vi "shared data GUI.vi"(0 "data update interval":refnum<vi>, 1 "Scroll Refnum":refnum<vi>, 5 "shared folder":refnum<vi>, 9 "My data to share":refnum<vi>, 11 "error in (no error)":errorcluster, 12 "command":enum16{"Initialize", "Update GUI"}(ring), 13 "Write":refnum<vi>, 14 "List of available data":refnum<vi>) -> (4 "Available shared data":T1 {"Shared Data"."scaled" format="%.2f"}, 6 "My data to share":T2 {"scaled" format="%.2f"}, 10 "Cumulative shared data sizes":i32[](array[numeric]), 15 "error out":errorcluster)   [LabVIEW 2015]
uses:
  shared data (name value unit).ctl
  available share data.ctl
  share data command.ctl
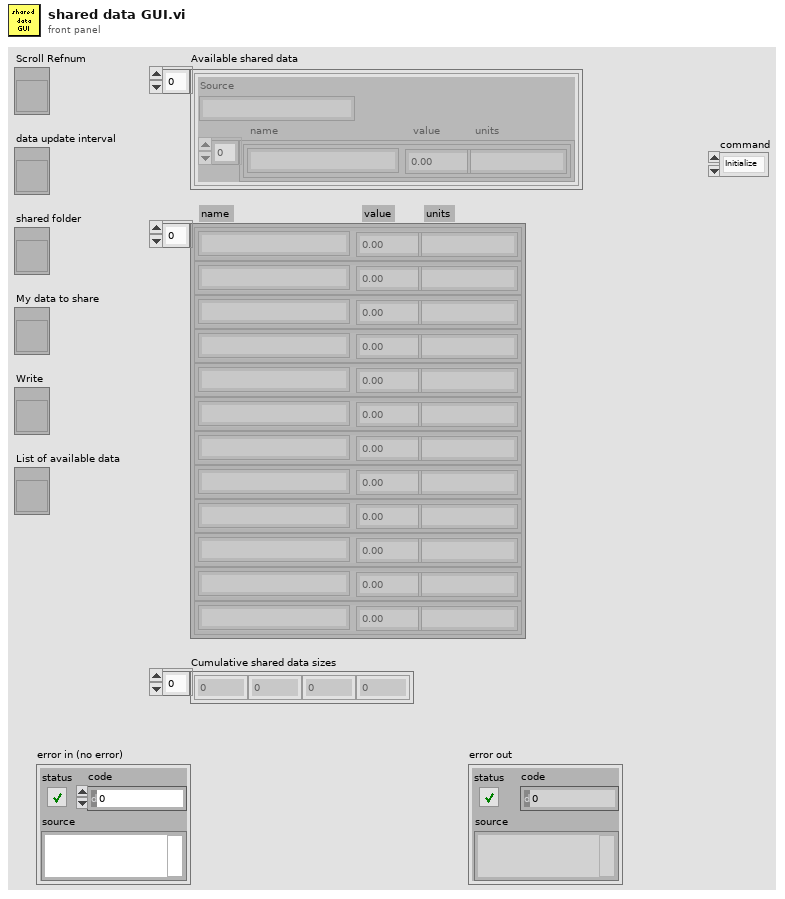
[diagram p1: front panel]
types:
  T1 = typedef "available share data.ctl" = cluster{"Source":string, "Shared Data":T2}[]
  T2 = typedef "shared data (name value unit).ctl" = cluster{"name":string, "units":string, "scaled":sgl}[]
  T3 = typedef "share data command.ctl" = enum16{"Initialize from ini", "Update ini", "Write data", "Read data", "List my data", "List shared data", "Close"}
  T4 = typedef "write data cluster.ctl" = cluster{"Data interval (s)":sgl, "Shared Folder":path, "Write":bool[]}
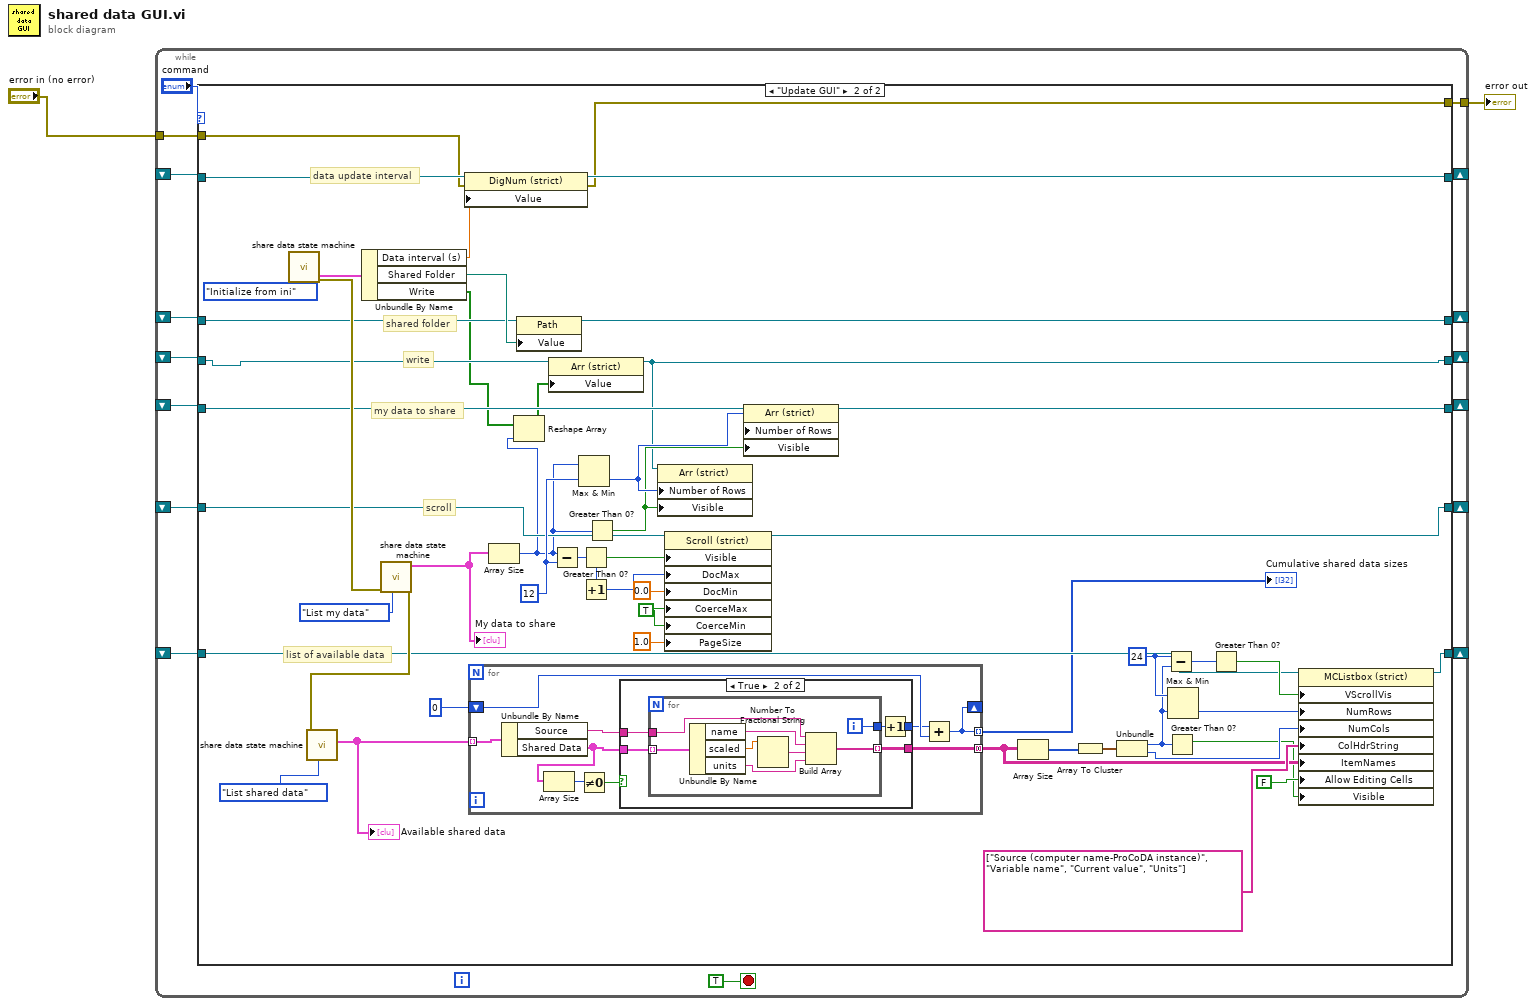
[diagram p0: block diagram]
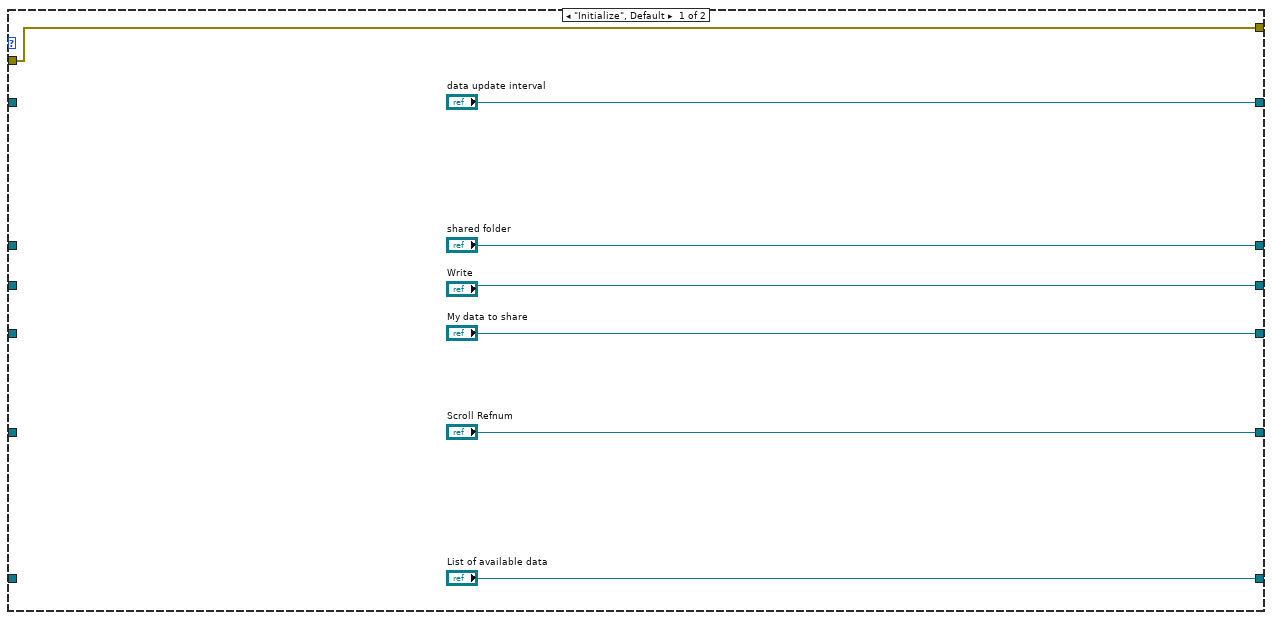
[diagram p2: hidden frame]
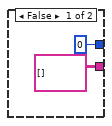
[diagram p3: hidden frame]
diagram:
  n1 = while {
    shift-right: [w16] -> _
    shift-left: _ -> [w11]
    shift-right: [w15] -> _
    shift-left: _ -> [w10]
    shift-right: [w13] -> _
    shift-left: _ -> [w9]
    shift-right: [w14] -> _
    shift-left: _ -> [w8]
    shift-right: [w17] -> _
    shift-left: _ -> [w7]
    shift-right: [w18] -> _
    shift-left: _ -> [w6]
    tunnel: "error in (no error)" -> [w4]
    tunnel: [w3] -> w1
    stop <- TRUE stop-if-true
    n2 = case shown="\"Update GUI\"" "command" {
      tunnel: ["My data to share" w34] -> w18
      tunnel: ["List of available data" w32] -> w17
      tunnel: ["data update interval" w37] -> w16
      tunnel: ["shared folder" w36] -> w15
      tunnel: ["Scroll Refnum" w33] -> w14
      tunnel: ["Write" w35] -> w13
      tunnel: w11 -> [_ w43]
      tunnel: w10 -> [_ w42]
      tunnel: w9 -> [_ w41]
      tunnel: w8 -> [_ w39]
      tunnel: w7 -> [_ w38]
      tunnel: w6 -> [_ w40]
      tunnel: w4 -> [w19 w31]
      tunnel: [w19 w30] -> w3
      frame "Initialize", Default {
      }
      frame "Update GUI" {
        w48 = 24 ("y")
        w55 = TRUE ("Coerce Maximum Value")
        w58 = 12 ("y")
        # "list of available data"
        # "scroll"
        # "my data to share"
        # "data update interval"
        # "shared folder"
        # "write"
        n3 = call "share data state machine.vi"("Share data command"=share_data_command."Initialize from ini") -> ("error out"=w73:errorcluster, "Write data cluster out"=w64:T4)  [unwired: 4 in, 5 out]
        n4 = Unbundle By Name(w64) -> ("Data interval (s)"=w63:sgl, "Shared Folder"=w62:path, "Write"=w27:bool[])
        n5 = call "share data state machine.vi"("Share data command"=share_data_command."List my data", "error in (no error)"=w73) -> ("error out"=w72:errorcluster, "My Data"=w70:T2)  [unwired: 3 in, 5 out]
        "My data to share" <- w70
        n6 = call "share data state machine.vi"("Share data command"=share_data_command."List shared data", "error in (no error)"=w72) -> ("Available shared data"=w69:T1)  [unwired: 3 in, 6 out]
        "Available shared data" <- w69
        n7 = property class="DigNum (strict)"(reference=w43, error in=w31, "Value"=w63) -> (reference out=w37:refnum<vi>, error out=w30:errorcluster)
        n8 = for {
          tunnel: w69 -> [w84] mode=indexing
          tunnel: [w82] -> w67 mode=concatenating
          shift-right: [w79] -> _
          shift-left: 0 -> [w81]
          tunnel: [w79] -> w29 mode=indexing
          n9 = Unbundle By Name(w84) -> ("Source"=w83:string, "Shared Data"=w78:T2)
          n10 = Array Size(array=w78) -> (size(s)=w77:i32)
          n11 = Not Equal To 0?(x=w77) -> (x != 0?=w76:bool)
          n12 = case shown="True" w76 {
            tunnel: w78 -> [_ w91]
            tunnel: w83 -> [_ w90]
            tunnel: [string[][] [] w89] -> w82
            tunnel: [0 w87] -> w80
            frame False {
            }
            frame True {
              n13 = for {
                tunnel: w91 -> [w99] mode=indexing
                tunnel: w90 -> [w97]
                tunnel: [w93] -> w89 mode=indexing
                tunnel: [w92] -> w88
                i -> [w92]
                n14 = Unbundle By Name(w99) -> ("name"=w96:string, "scaled"=w98:sgl, "units"=w94:string)
                n15 = Number To Fractional String(number=w98) -> (F-format string=w95:string)  [unwired: 3 in]
                n16 = Build Array(w97, w96, w95, w94) -> (w93:string[])
              }
              n17 = Increment(x=w88) -> (x+1=w87:i32)
            }
          }
          n18 = Add(x=w80, y=w81) -> (x+y=w79:i32)
        }
        "Cumulative shared data sizes" <- w29
        n19 = Array Size(array=w70) -> (size(s)=w28:i32)
        n20 = Reshape Array(w27, w28) -> (w26:bool[])
        n21 = property class="Path"(reference=w42, "Value"=w62) -> (reference out=w36:refnum<vi>)  [unwired: 1 in, 1 out]
        n22 = property class="Arr (strict)"(reference=w41, "Value"=w26) -> (reference out=w35:refnum<vi>)  [unwired: 1 in, 1 out]
        n23 = Subtract(x=w28, y=w58) -> (x-y=w50:i32)
        n24 = Max & Min(x=w28, y=w58) -> (min(x,y)=w57:i32)  [unwired: 1 out]
        n25 = Greater Than 0?(x=w50) -> (x > 0?=w49:bool)
        n26 = Increment(x=w50) -> (x+1=w53:i32)
        n27 = Greater Than 0?(x=w28) -> (x > 0?=w52:bool)
        n28 = property on="Property Node" class="Arr (strict)"(reference=w35, "Number of Rows"=w57, "Visible"=w52) -> ()  [unwired: 1 in, 2 out]
        n29 = property on="Property Node" class="Scroll (strict)"(reference=w39, "Visible"=w49, "DocMax"=w53, "DocMin"=0.0 ("Doc Min"), "CoerceMax"=w55, "CoerceMin"=w55, "PageSize"=1.0 ("Page Size")) -> (reference out=w33:refnum<vi>)  [unwired: 1 in, 1 out]
        n30 = property on="Property Node" class="Arr (strict)"(reference=w40, "Number of Rows"=w57, "Visible"=w52) -> (reference out=w34:refnum<vi>)  [unwired: 1 in, 1 out]
        n31 = Array Size(array=w67) -> (size(s)=w66:i32[])
        n32 = Array To Cluster(array=w66) -> (cluster=w65:cluster{"[0]":i32, "[1]":i32})
        n33 = Unbundle(w65) -> ("[0]"=w47:i32, "[1]"=w61:i32)
        n34 = Subtract(x=w48, y=w47) -> (x-y=w45:i32)
        n35 = Greater Than 0?(x=w47) -> (x > 0?=w51:bool)
        n36 = Max & Min(x=w48, y=w47) -> (min(x,y)=w46:i32)  [unwired: 1 out]
        n37 = Greater Than 0?(x=w45) -> (x > 0?=w44:bool)
        n38 = property on="Property Node" class="MCListbox (strict)"(reference=w38, "VScrollVis"=w44, "NumRows"=w46, "NumCols"=w61, "ColHdrString"=string[] ["Source (computer name-ProCoDA instance)", "Variable name", "Current value", "Units"] ("Row Header Strings[]"), "ItemNames"=w67, "Allow Editing Cells"=FALSE, "Visible"=w51) -> (reference out=w32:refnum<vi>)  [unwired: 1 in, 1 out]
      }
    }
  }
  "error out" <- w1
